vi "ConfirmRTMasterLoopRuning.vi"(8 "error in (no error)":errorcluster, 11 "CAlexVersion":T1=enum."Mobile") -> (0 "error out":errorcluster)   [LabVIEW 2016]
uses:
  Classes/CAlex2/TypeDef/CAlexVersion.ctl
  Classes/CAlex2/CAlex2.lvclass
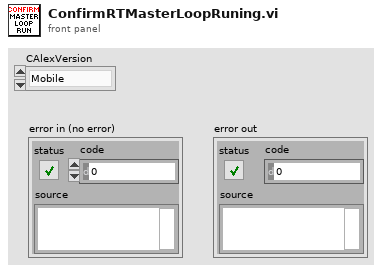
[diagram p1: front panel]
types:
  T1 = typedef "CAlex2.lvclass/CAlexVersion.ctl" = enum16{"Bilateral", "Squat", "Bilateral_Squat", "Treadmill", "Mobile"}
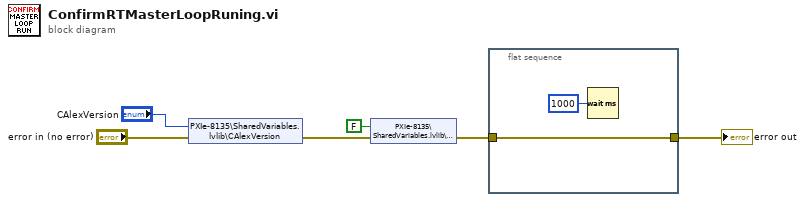
[diagram p0: block diagram]
diagram:
  n1 = shared-variable "PXIe-8135\\SharedVariables.lvlib\\CAlexVersion"("CAlexVersion", error in="error in (no error)") -> (error out=w3:errorcluster)
  n2 = shared-variable "PXIe-8135\\SharedVariables.lvlib\\Stop RT"(FALSE ("Stop RT"), error in=w3) -> (error out=w2:errorcluster)
  n3 = flat-sequence {
    tunnel: w2 -> [w8]
    tunnel: [w8] -> w1
    frame #0 {
      n4 = Wait (ms)(milliseconds to wait=u32 1000) -> ()  [unwired: 1 out]
    }
  }
  "error out" <- w1
